vi "Decimal String to Boolean.vi"(8 "error in (no error)":errorcluster, 11 "Excel Data":string[][](array[string])) -> (0 "error out":errorcluster, 3 "Boolean Data":bool[][](array[boolean]))   [LabVIEW 2021, in "User Interface.lvlib"]
uses:
  User Interface.lvlib
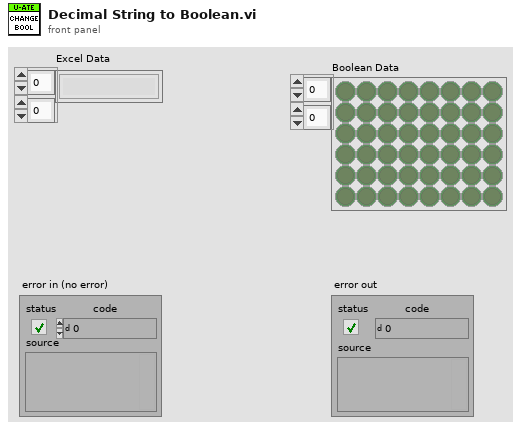
[diagram p1: front panel]
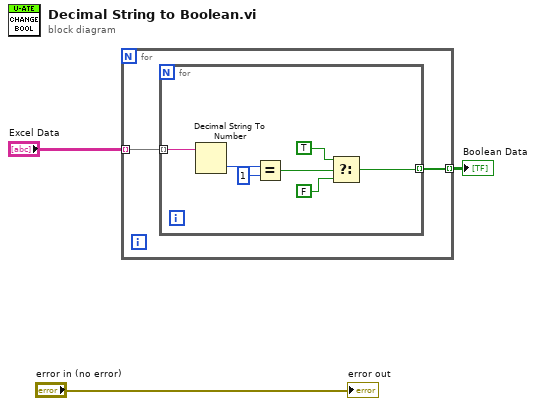
[diagram p0: block diagram]
diagram:
  n1 = for {
    tunnel: "Excel Data" -> [w5] mode=indexing
    tunnel: [w4] -> w1 mode=indexing
    n2 = for {
      tunnel: w5 -> [w12] mode=indexing
      tunnel: [w6] -> w4 mode=indexing
      n3 = Decimal String To Number(string=w12) -> (number=w11:i32)  [unwired: 2 in, 1 out]
      n4 = Equal?(x=w11, y=1) -> (x = y?=w9:bool)
      n5 = Select(t=TRUE, s=w9, f=FALSE) -> (s? t:f=w6:bool)
    }
  }
  "Boolean Data" <- w1
  "error out" <- "error in (no error)"
